vi "Check-Out.vi"(0 "File Data Manager in":refnum<class "File Data Manager.lvclass">, 5 "Room No":string, 11 "error in (no error)":errorcluster) -> (4 "File Data Manager out":refnum<class "File Data Manager.lvclass">, 15 "error out":errorcluster)   [LabVIEW 2023, in "File Data Manager.lvlib" / "File Data Manager.lvclass"]
uses:
  File Data Manager.lvclass
  C:/Program Files/National Instruments/LabVIEW 2023/vi.lib/ActorFramework/Actor/Actor.lvclass
  Database Selection.ctl
  File Data Manager.lvclass/File Data Manager.ctl
  Central Data Manager/Central Data Manager/Room Occupancy Status.ctl
  <vilib>/ActorFramework/Actor/Actor.lvclass/Actor.ctl
  <vilib>/ActorFramework/Message Enqueuer/Message Enqueuer.lvclass/Message Enqueuer.ctl
  Central Data Manager/Central Data Manager Messages/Write to Database Msg/Write to Database Msg.lvclass/Write to Database Msg.ctl
  <vilib>/ActorFramework/Message Enqueuer/Init from Existing Queue.vi
  <vilib>/ActorFramework/Message Enqueuer/Enqueue.vi
  Central Data Manager/Central Data Manager Messages/Refresh Rooms Status Msg/Refresh Rooms Status Msg.lvclass
  C:/Program Files/National Instruments/LabVIEW 2023/vi.lib/ActorFramework/Message/Message.lvclass
  Central Data Manager/Central Data Manager Messages/Write to Database Msg/Write to Database Msg.lvclass
  <vilib>/ActorFramework/Message Priority Queue/Priority Enqueue.vi
  <vilib>/ActorFramework/Message Enqueuer/Message Enqueuer.lvclass
  Central Data Manager/Central Data Manager/Central Data Manager.lvclass
  <vilib>/ActorFramework/Actor/Actor.lvclass
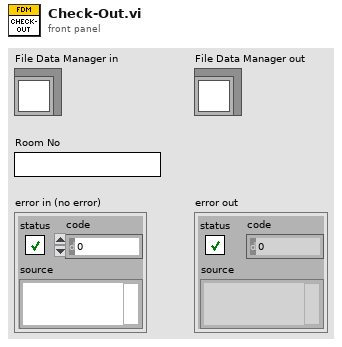
[diagram p1: front panel]
types:
  T1 = typedef "Central Data Manager.lvlib/Central Data Manager.lvclass/Room Occupancy Status.ctl" = enum16{"Not Occupied", "Occupied", "Under Maintainance", "Not Servicable"}
  T2 = typedef "Central Data Manager.lvlib/Central Data Manager.lvclass/Database Selection.ctl" = enum16{"Rooms List", "Guests History"}
  T3 = typedef "Central Data Manager.lvlib/Central Data Manager.lvclass/Room Details.ctl" = cluster{"Room No":string, "Room Size":string, "Room Occupancy Status":T1, "Guest Details":T4, "Occupancy Count (Adult)":u32, "Occupancy Count (Children)":u32, "Check-in Time":timestamp, "Check-out Time":timestamp}
  T4 = typedef "Central Data Manager.lvlib/Central Data Manager.lvclass/Guest Details.ctl" = cluster{"Contact Number":string, "Primary Guest Name":string}
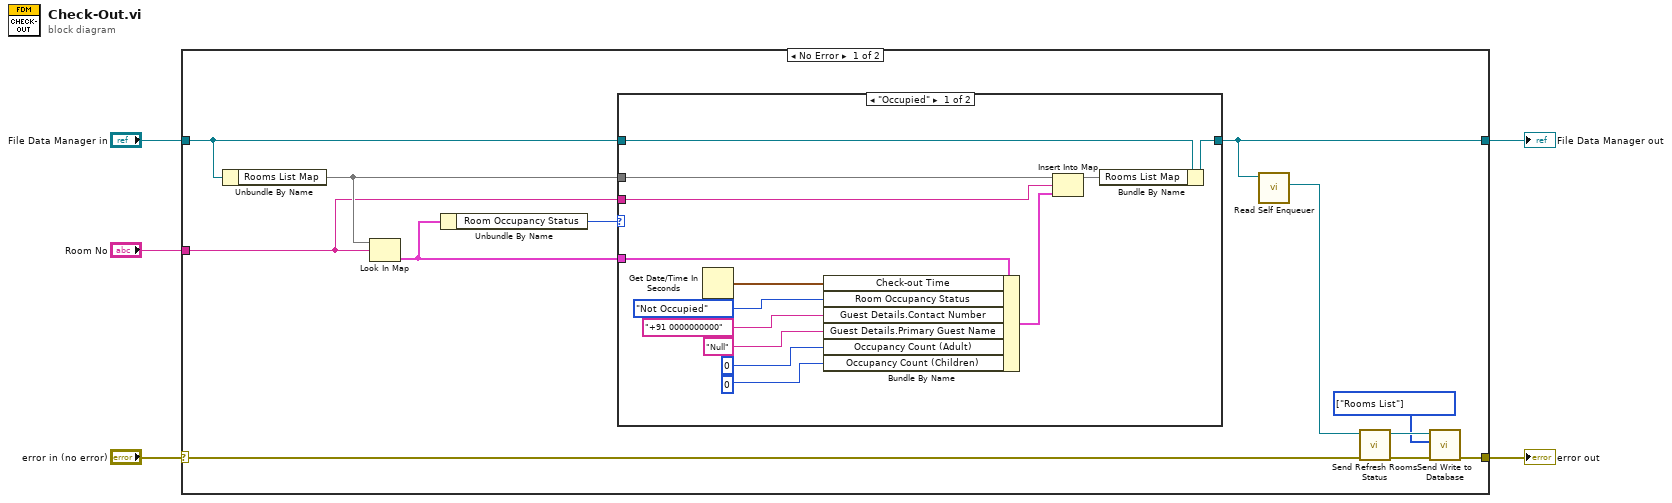
[diagram p0: block diagram]
diagram:
  n1 = case shown="No Error" "error in (no error)" {
    selector: "error in (no error)" -> [w13 w32]
    tunnel: "File Data Manager in" -> [w15 w33]
    tunnel: "Room No" -> [w10 _]
    tunnel: [w12 w33] -> w1
    tunnel: [w8 w32] -> w2
    frame No Error {
      w6 = T2[] [enum."Rooms List"] items=["Rooms List", "Guests History"] ("DB to Write")
      n2 = Unbundle By Name(w15) -> ("Rooms List Map"=w14:map{string, T3})
      n3 = Look In Map(map=w14, key=w10) -> (value=w16:T3)  [unwired: 1 in, 1 out]
      n4 = Unbundle By Name(w16) -> ("Room Occupancy Status"=w17:T1)
      n5 = case shown="\"Occupied\"" w17 {
        tunnel: w16 -> [w26 _]
        tunnel: w15 -> [w30 w31]
        tunnel: [w29 w31] -> w12
        tunnel: w14 -> [w28 _]
        tunnel: w10 -> [w22 _]
        frame "Occupied" {
          n6 = Get Date/Time In Seconds() -> (seconds since 1Jan1904=w24:timestamp)
          n7 = Bundle By Name(cluster=w26, "Check-out Time"=w24, "Room Occupancy Status"=Room_Occupancy_Status."Not Occupied", "Guest Details.Contact Number"="+91 0000000000", "Guest Details.Primary Guest Name"="Null", "Occupancy Count (Adult)"=u32 0, "Occupancy Count (Children)"=u32 0) -> (w23:T3)
          n8 = Insert Into Map(map in=w28, key=w22, value=w23) -> (map out=w27:map{string, T3})  [unwired: 2 out]
          n9 = Bundle By Name(cluster=w30, "Rooms List Map"=w27) -> (w29:refnum<class "File Data Manager.lvclass">)
        }
        frame Default {
        }
      }
      n10 = call <vilib>:"Read Self Enqueuer.vi"("Actor"=w12) -> ("Self Enqueuer"=w11:refnum<class "Message Enqueuer.lvclass">)  [unwired: 10 in]
      n11 = call "Send Refresh Rooms Status.vi"("error in (no error)"=w13, "Message Enqueuer"=w11) -> ("error out"=w9:errorcluster, "Message Enqueuer out"=w7:refnum<class "Message Enqueuer.lvclass">)  [unwired: 8 in]
      n12 = call "Send Write to Database.vi"("error in (no error)"=w9, "DB to Write"=w6, "Message Enqueuer"=w7) -> ("error out"=w8:errorcluster)  [unwired: 7 in, 1 out]
    }
    frame Error {
    }
  }
  "error out" <- w2
  "File Data Manager out" <- w1
